vi "Read Multiple - Wait On All.vi"(8 "error in (no error)":errorcluster, 9 "timeout in ms (60 sec)":i32=60000, 11 "Futures in":refnum<class "Future.lvclass">[](array[class])) -> (0 "error out":errorcluster, 1 "result error":errorcluster[](array[cluster]), 2 "Result value":variant[](array[variant]), 3 "Futures out":refnum<class "Future.lvclass">[](array[class]), 4 "timed out?":bool)   [LabVIEW 2017, in "Futures.lvlib" / "Future.lvclass"]
doc: "Read the result of the future.\n\nIf the future is resolved then the future becomes invalidated and cannot be read again.\n\nIf the future times out then you can attempt another read."
uses:
  Future.lvclass
  Future.lvclass/Future.ctl
  Result/Result.lvclass
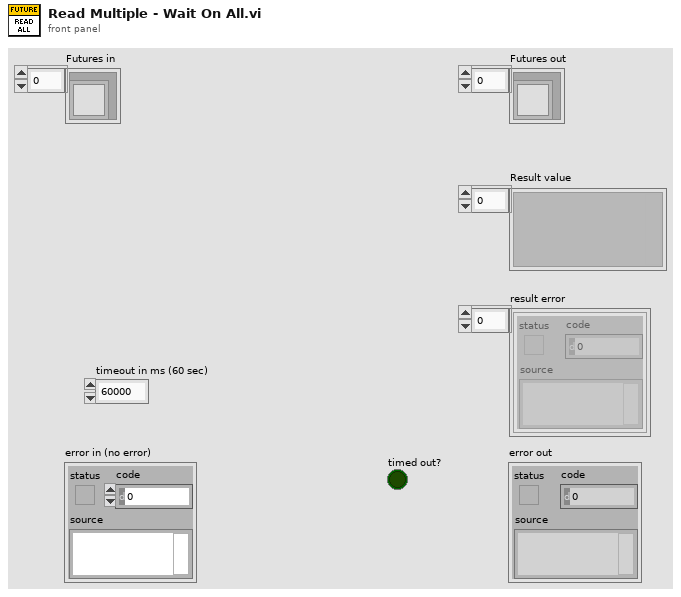
[diagram p1: front panel]
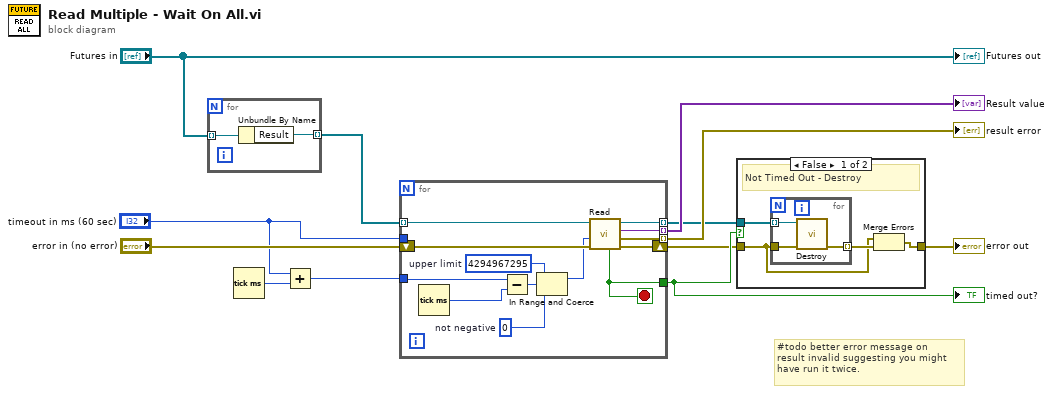
[diagram p0: block diagram]
diagram:
  # "#todo better error message on \nresult invalid suggesting you might\nhave run it twice."
  n1 = for {
    tunnel: "Futures in" -> [w14] mode=indexing
    tunnel: [w13] -> w6 mode=indexing
    n2 = Unbundle By Name(w14) -> ("Result"=w13:refnum<class "Result.lvclass">)
  }
  n3 = Tick Count (ms)() -> (millisecond timer value=w3:u32)
  n4 = Add(x="timeout in ms (60 sec)", y=w3) -> (x+y=w1:u32)
  n5 = for {
    tunnel: "timeout in ms (60 sec)" -> [_]
    tunnel: [w26] -> w9 mode=indexing
    tunnel: [w25] -> w8 mode=indexing
    tunnel: [w21] -> w7
    tunnel: w6 -> [w24] mode=indexing
    tunnel: [w22] -> w4 mode=indexing
    shift-right: [w23] -> w5
    shift-left: "error in (no error)" -> [w27]
    tunnel: w1 -> [w20]
    stop <- w21 stop-if-true
    w15 = u32 4294967295  # upper limit
    w16 = u32 0  # not negative
    n6 = Tick Count (ms)() -> (millisecond timer value=w19:u32)
    n7 = Subtract(x=w20, y=w19) -> (x-y=w18:u32)
    n8 = In Range and Coerce(upper limit=w15, x=w18, lower limit=w16) -> (coerced(x)=w17:u32)  [unwired: 1 out]
    n9 = call "Read.vi"("error in (no error)"=w27, "timeout in ms (-1)"=w17, "Result in"=w24) -> ("error out"=w23:errorcluster, "result error"=w25:errorcluster, "Result value"=w26:variant, "Result Out"=w22:refnum<class "Result.lvclass">, "timed out?"=w21:bool)  [unwired: 4 in]
  }
  "Result value" <- w9
  "result error" <- w8
  "timed out?" <- w7
  n10 = case shown="False" w7 {
    tunnel: w5 -> [w28 w35]
    tunnel: [w29 w35] -> w11
    tunnel: w4 -> [w30 _]
    frame False {
      # "Not Timed Out - Destroy"
      n11 = for {
        tunnel: w30 -> [w33] mode=indexing
        tunnel: w28 -> [w32]
        tunnel: [w34] -> w31 mode=indexing
        n12 = call "Destroy.vi"("error in (no error)"=w32, "Result in"=w33) -> ("error out"=w34:errorcluster)  [unwired: 9 in]
      }
      n13 = Merge Errors(w28, w31) -> (w29:errorcluster)
    }
    frame True {
      # "Timed Out - Keep for Repeat Attempt?"
    }
  }
  "error out" <- w11
  "Futures out" <- "Futures in"
